vi "ListDevice.vi"() -> (3 "Device Array":string[](array[string]))   [LabVIEW 2012, in "DeviceEnumXControl.xctl"]
uses:
  DeviceEnumXControl.xctl
  System.Management
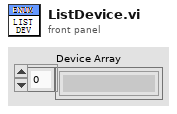
[diagram p1: front panel]
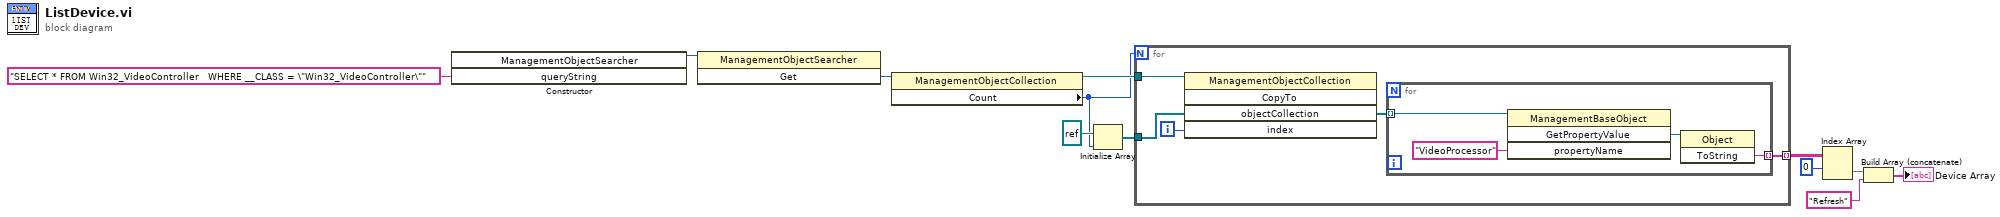
[diagram p0: block diagram]
diagram:
  n1 = constructor class="System.Management.ManagementObj"("queryString"="SELECT * FROM Win32_VideoController   WHERE __CLASS = \"Win32_VideoController\"") -> (reference out=w10:refnum<k24>)  [unwired: 3 in, 3 out]
  n2 = invoke class="ManagementObjectSearcher" method="Get"(reference=w10) -> ("Get"=w9:refnum<k24>)  [unwired: 2 in, 2 out]
  n3 = property class="ManagementObjectCollection"(reference=w9) -> (reference out=w8:refnum<k24>, "Count"=w6:i32)  [unwired: 1 in, 1 out]
  n4 = Initialize Array(refnum<k24> refnum, w6) -> (w5:refnum<k24>[])
  n5 = for {
    N: w6 -> [_]
    tunnel: w8 -> [w17]
    tunnel: w5 -> [w16]
    tunnel: [w13] -> w3 mode=indexing
    i -> [w15]
    n6 = invoke class="ManagementObjectCollection" method="CopyTo"(reference=w17, "objectCollection"=w16, "index"=w15) -> ("objectCollection"=w14:refnum<k24>[])  [unwired: 2 in, 4 out]
    n7 = for {
      tunnel: w14 -> [w21] mode=indexing
      tunnel: [w18] -> w13 mode=indexing
      n8 = invoke class="ManagementBaseObject" method="GetPropertyValue"(reference=w21, "propertyName"="VideoProcessor") -> ("GetPropertyValue"=w19:refnum<k24>)  [unwired: 2 in, 3 out]
      n9 = invoke class="Object" method="ToString"(reference=w19) -> ("ToString"=w18:string)  [unwired: 2 in, 2 out]
    }
  }
  n10 = Index Array(array=w3, index (row)=0 ("dimension size")) -> (element=w2:string[])  [unwired: 1 in]
  n11 = Build Array (concatenate)(w2, "Refresh") -> (→"Device Array":string[])
